vi "onSubscribe.vi"(6 "timeout (100ms)":i32=100, 8 "error in (no error)":errorcluster, 10 "SUBSCRIBE":refnum<class "SUBSCRIBE.lvclass">, 11 "Client in":refnum<class "Client.lvclass">) -> (0 "error out":errorcluster, 1 "Ack?":bool, 2 "SUBACK":refnum<class "SUBACK.lvclass">, 3 "Client out":refnum<class "Client.lvclass">)   [LabVIEW 2013, in "MQTT Client.lvlib" / "Client.lvclass"]
uses:
  Client.lvclass
  <vilib>/LabVIEW Open Source Project/MQTT Control Packets/Control Packets/SUBSCRIBE/SUBSCRIBE.lvclass
  <vilib>/LabVIEW Open Source Project/MQTT Control Packets/Control Packets/SUBACK/SUBACK.lvclass
  <vilib>/LabVIEW Open Source Project/MQTT Control Packets/Control Packets/ControlPacket/ControlPacket.lvclass/ControlPacket.ctl
  MQTT_Base/Base Class/MQTT_Base.lvclass
  Client.lvclass/Client.ctl
  Session.Client/Session.Client.lvclass
  <vilib>/LabVIEW Open Source Project/MQTT Control Packets/Control Packets/ControlPacket/ControlPacket.lvclass
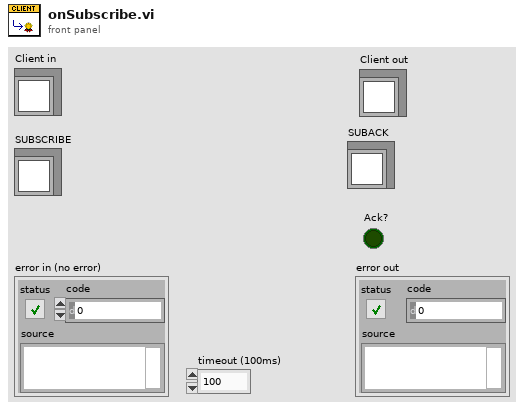
[diagram p1: front panel]
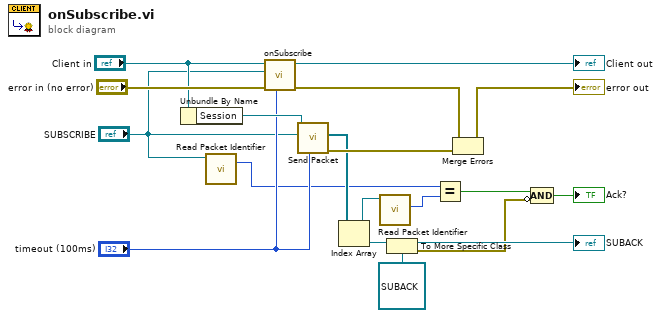
[diagram p0: block diagram]
diagram:
  n1 = Unbundle By Name("Client in") -> ("Session"=w15:refnum<class "Session.Client.lvclass">)
  n2 = call <vilib>:"Read Packet Identifier.vi"("ControlPacket in"="SUBSCRIBE") -> ("Packet Identifier"=w4:u16)  [unwired: 9 in, 1 out]
  n3 = call-parent "onSubscribe.vi"("timeout (100ms)"="timeout (100ms)", "error in (no error)"="error in (no error)", "SUBSCRIBE"="SUBSCRIBE", "MQTT_Base in"="Client in") -> ("error out"=w13:errorcluster, "MQTT_Base out"=→"Client out":refnum<class "Client.lvclass">)  [unwired: 4 in, 2 out]
  n4 = call "Send Packet.vi"("timeout (0ms : no ack)"="timeout (100ms)", "Packet"="SUBSCRIBE", "Session"=w15) -> ("error out"=w14:errorcluster, "Response"=w10:refnum<class "ControlPacket.lvclass">[])  [unwired: 5 in, 2 out]
  n5 = Index Array(array=w10) -> (element=w6:refnum<class "ControlPacket.lvclass">)  [unwired: 1 in]
  n6 = call <vilib>:"Read Packet Identifier.vi"("ControlPacket in"=w6) -> ("Packet Identifier"=w5:u16)  [unwired: 9 in, 1 out]
  n7 = To More Specific Class(target class=refnum<class "SUBACK.lvclass"> refnum ("SUBACK.lvclass"), reference=w6) -> (specific class reference=→"SUBACK":refnum<class "SUBACK.lvclass">, error out=w2:errorcluster)  [unwired: 1 in]
  n8 = Equal?(x=w4, y=w5) -> (x = y?=w3:bool)
  n9 = Merge Errors(w13, w14) -> (→"error out":errorcluster)
  n10 = Compound Arithmetic op=AND(w3, invert w2) -> (→"Ack?":bool)
